vi "1.3.16 New What.vi"() -> ()   [LabVIEW 2010]
uses:
  Lidar Test Global.vi
  1.0-Hindbrain Global.vi
panel:
  out "ReadBit":bool
  out "Write Bitarray":bool[](array[boolean])
  out "Write Counter Outer":u16
  out "Bitarray":bool[](array[boolean])
  out "Transmission Error":bool
  out "Other Inner Loop Counter":u8
  out "Went Through":bool
  out "Transmit":u16
  out "Counter Outer":u16
  out "Counter Inner":u16
  out "Test Val":u16
  out "Angle":u8
  out "Magnitude":u16
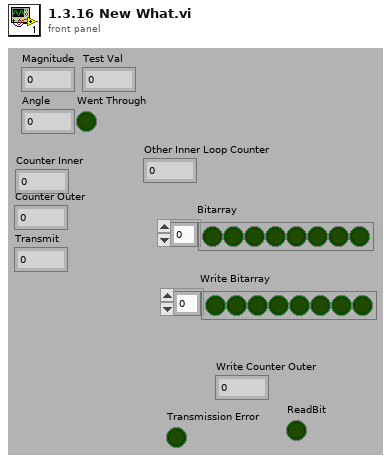
[diagram p1: front panel]
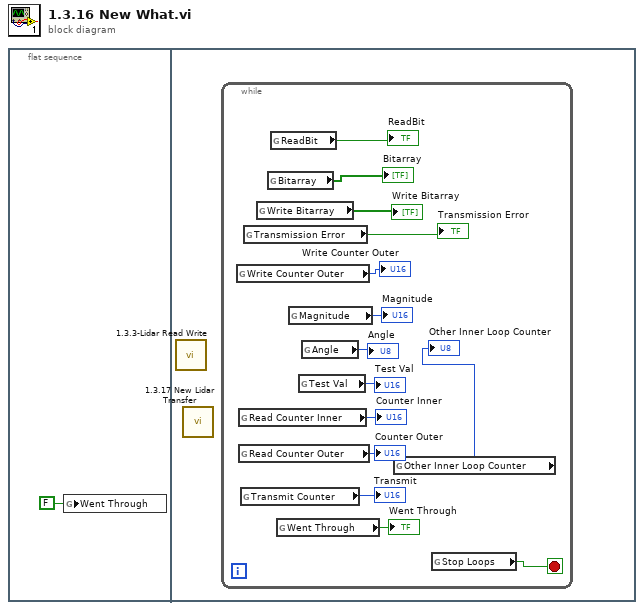
[diagram p0: block diagram]
diagram:
  n1 = flat-sequence {
    frame #0 {
      n2 = global write "Lidar Test Global.vi" "Went Through"(FALSE ("Went Through")) -> ()
    }
    frame #1 {
      n3 = call "1.3.3-Lidar Read Write.vi"() -> ()  [unwired: 1 in]
      n4 = call "1.3.17 New Lidar Transfer.vi"() -> ()  [unwired: 12 in]
      n5 = while {
        stop <- w15 stop-if-true
        n6 = global read "Lidar Test Global.vi" "Write Counter Outer"() -> (→"Write Counter Outer":u16)
        n7 = global read "Lidar Test Global.vi" "Read Counter Inner"() -> (→"Counter Inner":u16)
        n8 = global read "Lidar Test Global.vi" "Read Counter Outer"() -> (→"Counter Outer":u16)
        n9 = global read "Lidar Test Global.vi" "Transmit Counter"() -> (→"Transmit":u16)
        n10 = global read "Lidar Test Global.vi" "Transmission Error"() -> (→"Transmission Error":bool)
        n11 = global read "Lidar Test Global.vi" "Write Bitarray"() -> (→"Write Bitarray":bool[])
        n12 = global read "Lidar Test Global.vi" "Bitarray"() -> (→"Bitarray":bool[])
        n13 = global read "Lidar Test Global.vi" "ReadBit"() -> (→"ReadBit":bool)
        n14 = global read "Lidar Test Global.vi" "Went Through"() -> (→"Went Through":bool)
        n15 = global read "Lidar Test Global.vi" "Magnitude"() -> (→"Magnitude":u16)
        n16 = global read "Lidar Test Global.vi" "Test Val"() -> (→"Test Val":u16)
        n17 = global read "Lidar Test Global.vi" "Angle"() -> (→"Angle":u8)
        n18 = global read "Lidar Test Global.vi" "Other Inner Loop Counter"() -> (→"Other Inner Loop Counter":u8)
        n19 = global read "1.0-Hindbrain Global.vi" "Stop Loops"() -> (w15:bool)
      }
    }
  }
